vi "Vision Processing.vi"(4 "error in (no error)":errorcluster, 7 "Image Size":T1=enum."320x240") -> ()   [LabVIEW 2016]
doc: "This VI runs in parallel to other tasks. It gets images from the camera, processes them for color or shape and uses commands or globals to affect the behavior of other subsystems."
uses:
  <vilib>/Rock Robotics/WPI/Camera/WPI_CameraImageSize.ctl
  <vilib>/Rock Robotics/WPI/Camera/WPI_CameraWhite Balance Values.ctl
  <vilib>/Rock Robotics/WPI/Camera/WPI_CameraExposure Values.ctl
  <vilib>/Rock Robotics/WPI/Camera/WPI_CameraFrameRate.ctl
  Framework/Robot Global Data.vi
  Drive/Implementation/Drive Published Globals.vi
  <vilib>/Rock Robotics/Network Tables/NT Read Numeric Array.vi
  <vilib>/Rock Robotics/Network Tables/NT Write Number.vi
  <vilib>/Rock Robotics/Network Tables/NT Write Numeric Array.vi
  <vilib>/vision/NI_Vision_Development_Module.lvlib
panel:
  in  "Brightness":i32=20
  in  "Score Cutoff %":dbl=70.0
  in  "Particle Count Limit":dbl=inf
  out "Qualified Particles":i32=2
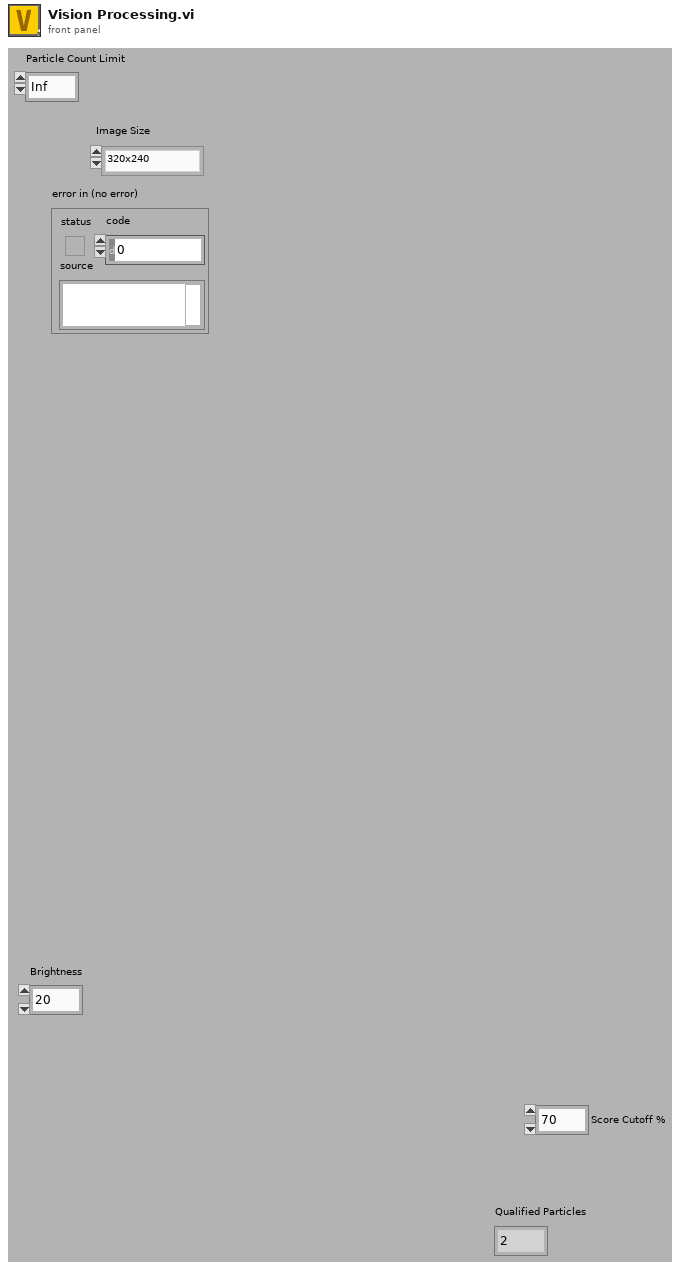
[diagram p1: front panel]
types:
  T1 = typedef "WPI_CameraImageSize.ctl" = enum16{"640x480", "320x240", "160x120", "Custom"}
  T2 = typedef "Image Type" = u32
  T3 = typedef "WPI_CameraFrameRate.ctl" = u32
  T4 = typedef "WPI_CameraExposure Values.ctl" = enum16{"Auto", "Flicker-free 50 Hz", "Flicker-free 60 Hz", "Hold current", "Custom"}
  T5 = typedef "WPI_CameraWhite Balance Values.ctl" = enum16{"Auto", "Fixed indoor", "Fixed outdoor 1", "Fixed outdoor 2", "Fixed fluorescent 1", "Fixed fluorescent 2", "Hold current", "Custom"}
  T6 = typedef "WPI_CameraDevRef.ctl" = cluster{"Camera Address":string, "CameraStatus":errorcluster}
  T7 = typedef "IMAQ Image.ctl" = refnum<image>
  T8 = cluster{"Left":dbl, "Top":dbl, "Right":dbl, "Bottom":dbl}
  T9 = typedef "Particle Parameters" = i32
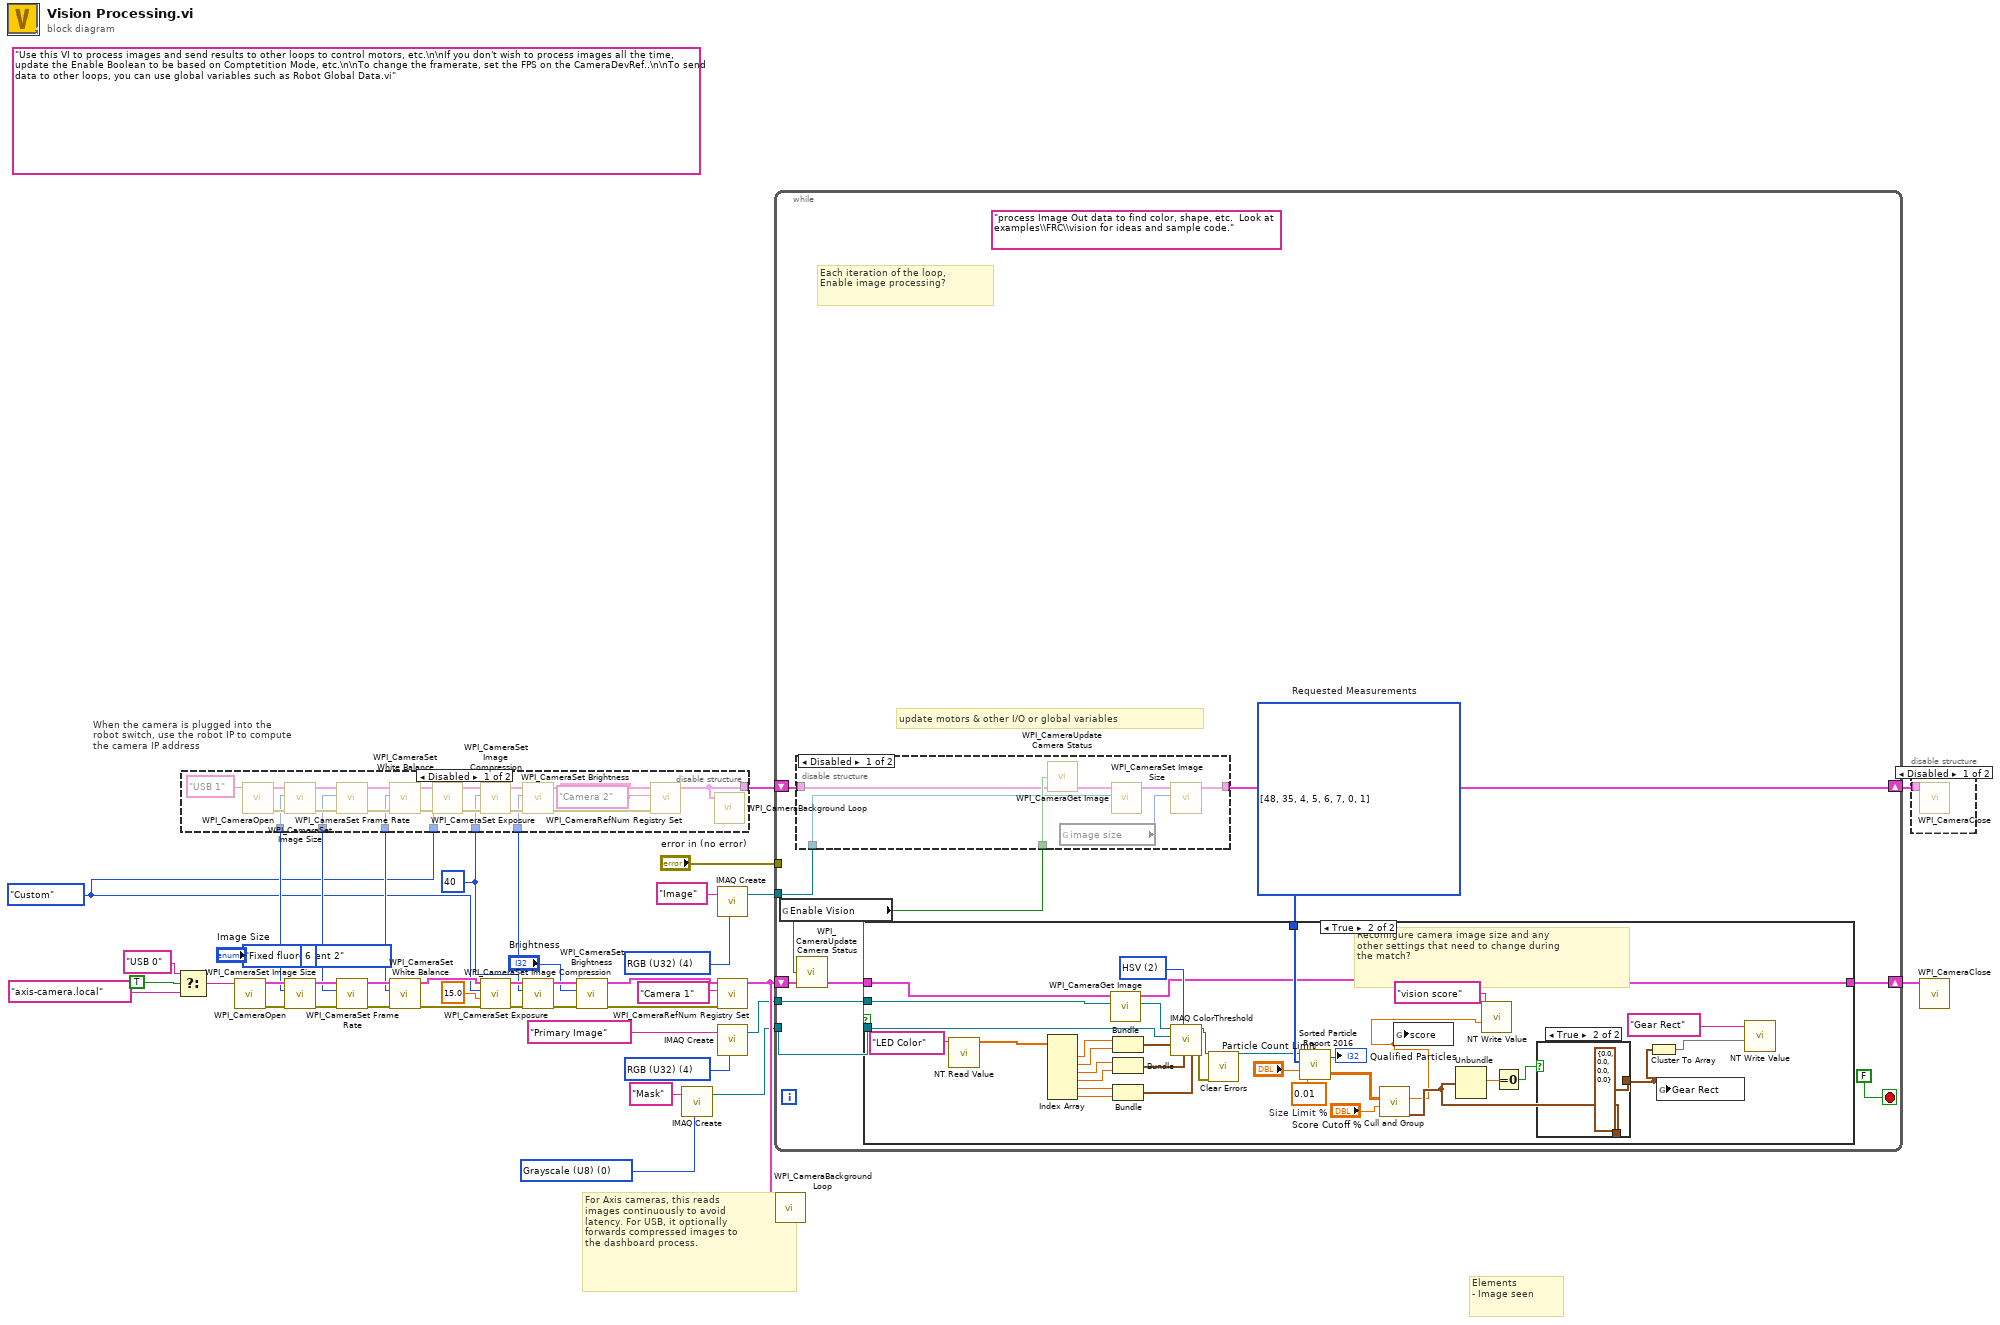
[diagram p0: block diagram]
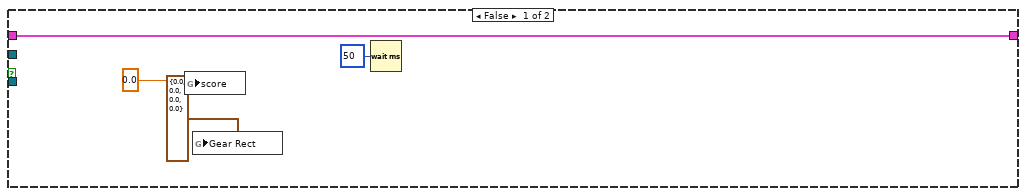
[diagram p4: hidden frame]
diagram:
  w3 = T2 0 items=["Grayscale (U8)", "Grayscale (I16)", "Grayscale (SGL)", "Complex (CSG)", "RGB (U32)", "HSL (U32)", "RGB (U64)", "Grayscale (U16)"] ("Image Type")
  w7 = T2 4 items=["Grayscale (U8)", "Grayscale (I16)", "Grayscale (SGL)", "Complex (CSG)", "RGB (U32)", "HSL (U32)", "RGB (U64)"] ("Image Type")
  w15 = T3 6 ("Frame Rate (fps)")
  w13 = WPI_CameraExposure_Values."Custom" ("Exposure")
  w14 = WPI_CameraWhite_Balance_Values."Fixed fluorescent 2" ("White Balance")
  w12 = 40 ("Compression")
  (unwired) "Use this VI to process images and send results to other loops to control motors, etc.\n\nIf you don't wish to process images all the time, update the Enable Boolean to be based on Comptetition Mode, etc.\n\nTo change the framerate, set the FPS on the CameraDevRef..\n\nTo send data to other loops, you can use global variables such as Robot Global Data.vi"
  w40 = T2 4 items=["Grayscale (U8)", "Grayscale (I16)", "Grayscale (SGL)", "Complex (CSG)", "RGB (U32)", "HSL (U32)", "RGB (U64)"] ("Image Type")
  # "Elements\n- Image seen"
  # "When the camera is plugged into the\nrobot switch, use the robot IP to compute\nthe camera IP address"
  # "For Axis cameras, this reads\nimages continuously to avoid\nlatency. For USB, it optionally\nforwards compressed images to\nthe dashboard process."
  n1 = Select(t="USB 0" ("format string"), s=TRUE ("dot notation? (F)"), f="axis-camera.local" ("format string")) -> (s? t:f=w18:string)
  n2 = disable-structure shown="Disabled" {
    disable-tunnel: "Image Size" -> [w48 _]
    disable-tunnel: w15 -> [w47 _]
    disable-tunnel: w14 -> [w46 _]
    disable-tunnel: w13 -> [w45 _]
    disable-tunnel: w12 -> [w44 _]
    disable-tunnel: "Brightness" -> [w43 _]
    disable-tunnel: [w41 _] -> w5
    frame Disabled {
      n3 = call <vilib>:"WPI_CameraOpen.vi"("Camera Address"="USB 1") -> ("error out"=w61:errorcluster, "CameraDevRef"=w62:T6)  [unwired: 2 in, 7 out]
      n4 = call <vilib>:"WPI_CameraSet Image Size.vi"("error in (no error)"=w61, "Image Size"=w48, "CameraDevRef"=w62) -> ("error out"=w54:errorcluster, "CameraDevRef Out"=w60:T6)  [unwired: 1 in, 6 out]
      n5 = call <vilib>:"WPI_CameraSet Frame Rate.vi"("error in (no error)"=w54, "Frame Rate (fps)"=w47, "CameraDevRef"=w60) -> ("error out"=w53:errorcluster, "CameraDevRef Out"=w59:T6)  [unwired: 7 out]
      n6 = call <vilib>:"WPI_CameraSet White Balance.vi"("error in (no error)"=w53, "White Balance"=w46, "CameraDevRef"=w59) -> ("error out"=w52:errorcluster, "CameraDevRef Out"=w58:T6)  [unwired: 1 in, 6 out]
      n7 = call <vilib>:"WPI_CameraSet Exposure.vi"("error in (no error)"=w52, "Exposure"=w45, "CameraDevRef"=w58) -> ("error out"=w51:errorcluster, "CameraDevRef Out"=w57:T6)  [unwired: 1 in, 6 out]
      n8 = call <vilib>:"WPI_CameraSet Image Compression.vi"("error in (no error)"=w51, "Compression"=w44, "CameraDevRef"=w57) -> ("error out"=w50:errorcluster, "CameraDevRef Out"=w56:T6)  [unwired: 7 out]
      n9 = call <vilib>:"WPI_CameraSet Brightness.vi"("error in (no error)"=w50, "Brightness"=w43, "CameraDevRef"=w56) -> ("error out"=w49:errorcluster, "CameraDevRef Out"=w55:T6)  [unwired: 7 out]
      n10 = call <vilib>:"WPI_CameraRefNum Registry Set.vi"("error in (no error)"=w49, "refnum name"="Camera 2", "CameraDevRef"=w55) -> ("CameraDevRef"=w41:T6)  [unwired: 1 in, 7 out]
      n11 = call <vilib>:"WPI_CameraBackground Loop.vi"("CameraDevRef"=w41) -> ()  [unwired: 11 in]
    }
    frame Enabled {
    }
  }
  n12 = call <vilib>:"WPI_CameraOpen.vi"("Camera Address"=w18) -> ("error out"=w31:errorcluster, "CameraDevRef"=w32:T6)  [unwired: 2 in, 7 out]
  n13 = call <vilib>:"WPI_CameraSet Image Size.vi"("error in (no error)"=w31, "Image Size"="Image Size", "CameraDevRef"=w32) -> ("error out"=w30:errorcluster, "CameraDevRef Out"=w33:T6)  [unwired: 1 in, 6 out]
  n14 = call <vilib>:"WPI_CameraSet Frame Rate.vi"("error in (no error)"=w30, "Frame Rate (fps)"=w15, "CameraDevRef"=w33) -> ("error out"=w29:errorcluster, "CameraDevRef Out"=w35:T6)  [unwired: 7 out]
  n15 = call <vilib>:"WPI_CameraSet White Balance.vi"("error in (no error)"=w29, "White Balance"=w14, "CameraDevRef"=w35) -> ("error out"=w28:errorcluster, "CameraDevRef Out"=w34:T6)  [unwired: 1 in, 6 out]
  n16 = call <vilib>:"WPI_CameraSet Exposure.vi"("error in (no error)"=w28, "Exposure (%)"=15.0, "Exposure"=w13, "CameraDevRef"=w34) -> ("error out"=w27:errorcluster, "CameraDevRef Out"=w37:T6)  [unwired: 6 out]
  n17 = call <vilib>:"WPI_CameraSet Image Compression.vi"("error in (no error)"=w27, "Compression"=w12, "CameraDevRef"=w37) -> ("error out"=w26:errorcluster, "CameraDevRef Out"=w36:T6)  [unwired: 7 out]
  n18 = call <vilib>:"WPI_CameraSet Brightness.vi"("error in (no error)"=w26, "Brightness"="Brightness", "CameraDevRef"=w36) -> ("error out"=w24:errorcluster, "CameraDevRef Out"=w25:T6)  [unwired: 7 out]
  n19 = call "IMAQ Create"("Image Name"="Mask", "Image Type"=w3) -> ("New Image"=w1:T7)  [unwired: 2 in, 2 out]
  n20 = call "IMAQ Create"("Image Name"="Image", "Image Type"=w7) -> ("New Image"=w6:T7)  [unwired: 2 in, 2 out]
  n21 = call <vilib>:"WPI_CameraRefNum Registry Set.vi"("error in (no error)"=w24, "refnum name"="Camera 1", "CameraDevRef"=w25) -> ("CameraDevRef"=w23:T6)  [unwired: 1 in, 7 out]
  n22 = call "IMAQ Create"("Image Name"="Primary Image", "Image Type"=w40) -> ("New Image"=w10:T7)  [unwired: 2 in, 2 out]
  n23 = while {
    shift-right: [w73] -> w22
    shift-left: w23 -> [w71]
    tunnel: w10 -> [w72]
    tunnel: "error in (no error)" -> [_]
    tunnel: w6 -> [w69]
    shift-right: [w68] -> w9
    shift-left: w5 -> [w67]
    tunnel: w1 -> [w66]
    stop <- FALSE stop-if-true
    w64 = T9[] [48, 35, 4, 5, 6, 7, 0, 1] items=["Center of Mass X", "Center of Mass Y", "First Pixel X", "First Pixel Y", "Bounding Rect Left", "Bounding Rect Top", "Bounding Rect Right", "Bounding Rect Bottom", "Max Feret Diameter Start X", "Max Feret Diameter Start Y", "Max Feret Diameter End X", "Max Feret Diameter End Y", "Max Horiz. Segment Length Left", "Max Horiz. Segment Length Right", "Max Horiz. Segment Length Row", "-", "Bounding Rect Width", "Bounding Rect Height", "Bounding Rect Diagonal", "Perimeter", "Convex Hull Perimeter", "Holes' Perimeter", "Max Feret Diameter", "Equivalent Ellipse Major Axis", "Equivalent Ellipse Minor Axis", "Equivalent Ellipse Minor Axis (Feret)", "Equivalent Rect Long Side", "Equivalent Rect Short Side", "Equivalent Rect Diagonal", "Equivalent Rect Short Side (Feret)", "Average Horiz. Segment Length", "Average Vert. Segment Length", "Hydraulic Radius", "Waddel Disk Diameter", "-", "Area", "Holes' Area", "Particle & Holes' Area", "Convex Hull Area", "Image Area", "-", "Number of Holes", "Number of Horiz. Segments", "Number of Vert. Segments", "-", "Orientation", "Max Feret Diameter Orientation", "-", "% Area/Image Area", "% Area/(Particle & Holes' Area)", "Ratio of Equivalent Ellipse Axes", "Ratio of Equivalent Rect Sides", "-", "Elongation Factor", "Compactness Factor", "Heywood Circularity Factor", "Type Factor", "-", "Sum X", "Sum Y", "Sum XX", "Sum XY", "Sum YY", "Sum XXX", "Sum XXY", "Sum XYY", "Sum YYY", "-", "Moment of Inertia XX", "Moment of Inertia XY", "Moment of Inertia YY", "Moment of Inertia XXX", "Moment of Inertia XXY", "Moment of Inertia XYY", "Moment of Inertia YYY", "Norm. Moment of Inertia XX", "Norm. Moment of Inertia XY", "Norm. Moment of Inertia YY", "Norm. Moment of Inertia XXX", "Norm. Moment of Inertia XXY", "Norm. Moment of Inertia XYY", "Norm. Moment of Inertia YYY", "Hu Moment 1", "Hu Moment 2", "Hu Moment 3", "Hu Moment 4", "Hu Moment 5", "Hu Moment 6", "Hu Moment 7"]  # Requested Measurements
    (unwired) "process Image Out data to find color, shape, etc.  Look at examples\\FRC\\vision for ideas and sample code."
    # "update motors & other I/O or global variables"
    # "Each iteration of the loop,\nEnable image processing?"
    n24 = global read "Robot Global Data.vi" "Enable Vision"() -> (w65:bool)
    n25 = disable-structure shown="Disabled" {
      disable-tunnel: w65 -> [w120 _]
      disable-tunnel: w69 -> [w118 _]
      disable-tunnel: [w117 _] -> w68
      disable-tunnel: w67 -> [w116 _]
      frame Disabled {
        n26 = call <vilib>:"WPI_CameraUpdate Camera Status.vi"("CameraDevRef In"=w116, "Enable Vision"=w120) -> ("CameraDevRef Out"=w119:T6)  [unwired: 3 in]
        n27 = global read "Robot Global Data.vi" "image size"() -> (w115:T1)
        n28 = call <vilib>:"WPI_CameraGet Image.vi"("Image"=w118, "CameraDevRef"=w119) -> ("CameraDevRef Out"=w114:T6)  [unwired: 1 in, 8 out]
        n29 = call <vilib>:"WPI_CameraSet Image Size.vi"("Image Size"=w115, "CameraDevRef"=w114) -> ("CameraDevRef Out"=w117:T6)  [unwired: 2 in, 7 out]
      }
      frame Enabled {
      }
    }
    n30 = call <vilib>:"WPI_CameraUpdate Camera Status.vi"("CameraDevRef In"=w71, "Enable Vision"=w65) -> ("CameraDevRef Out"=w70:T6)  [unwired: 3 in]
    n31 = case shown="True" w65 {
      tunnel: [w78 w83] -> w73
      tunnel: w72 -> [_ w111]
      tunnel: w70 -> [w78 w110]
      tunnel: w66 -> [_ w108]
      tunnel: w64 -> [_ w91]
      frame False {
        n32 = global write "Drive Published Globals.vi" "score"(0.0) -> ()
        n33 = global write "Drive Published Globals.vi" "Gear Rect"(T8 {"Left"=0.0, "Top"=0.0, "Right"=0.0, "Bottom"=0.0} ("Gear Rect")) -> ()
        n34 = Wait (ms)(milliseconds to wait=u32 50) -> ()  [unwired: 1 out]
      }
      frame True {
        w92 = u16 2 items=["RGB", "HSL", "HSV", "HSI"] ("Color Mode")
        w95 = 0.01  # Size Limit %
        # "Reconfigure camera image size and any\nother settings that need to change during\nthe match?"
        n35 = call-poly <vilib>:"NT Read Value.vi"("Name"="LED Color") -> ("Numeric Array"=w106:dbl[])  [unwired: 9 in, 1 out]
        n36 = Index Array(array=w106) -> (element #1=w104:dbl, element #2=w105:dbl, element #3=w103:dbl, element #4=w102:dbl, element #5=w101:dbl, element #6=w100:dbl)  [unwired: 6 in]
        n37 = call <vilib>:"WPI_CameraGet Image.vi"("Image"=w111, "CameraDevRef"=w110) -> ("Image Out"=w109:T7, "CameraDevRef Out"=w83:T6)  [unwired: 1 in, 7 out]
        n38 = Bundle("Numeric"=w104, "Numeric"=w105) -> (w99:cluster{"Numeric":dbl, "Numeric":dbl})  [unwired: 1 in]
        n39 = Bundle("Numeric"=w103, "Numeric"=w102) -> (w98:cluster{"Numeric":dbl, "Numeric":dbl})  [unwired: 1 in]
        n40 = Bundle("Numeric"=w101, "Numeric"=w100) -> (w97:cluster{"Numeric":dbl, "Numeric":dbl})  [unwired: 1 in]
        n41 = call "IMAQ ColorThreshold"("Blue or Luma or Val or Inten Range"=w97, "Green or Sat Range"=w98, "Color Mode"=w92, "Red or Hue Range"=w99, "Image Dst"=w108, "Image Src"=w109) -> ("error out"=w96:errorcluster, "Image Dst Out"=w87:T7)  [unwired: 4 in]
        n42 = call <vilib>:"Clear Errors.vi"("error in (no error)"=w96) -> ()  [unwired: 5 in, 2 out]
        n43 = call "Sorted Particle Report 2016.vi"("Min Area Size %"=w95, "Particle Count Limit"="Particle Count Limit", "Pixel Measurements"=w91, "Image in"=w87) -> ("Sorted Data"=w81:dbl[][], "Particles"=→"Qualified Particles":i32)
        n44 = call "Cull and Group.vi"("Score Cutoff"="Score Cutoff %", "Sorted Data"=w81) -> ("Rect"=w80:T8, "Score"=w79:dbl)  [unwired: 6 in, 2 out]
        n45 = global write "Drive Published Globals.vi" "score"(w79) -> ()
        n46 = Unbundle(w80) -> ("Top"=w89:dbl)  [unwired: 3 out]
        n47 = call-poly <vilib>:"NT Write Value.vi"("Numeric"=w79, "Name"="vision score") -> ()  [unwired: 9 in, 1 out]
        n48 = Equal To 0?(x=w89) -> (x = 0?=w88:bool)
        n49 = case shown="True" w88 {
          tunnel: [w112 T8 {"Left"=0.0, "Top"=0.0, "Right"=0.0, "Bottom"=0.0} ("Rect")] -> w86
          tunnel: w80 -> [w112 _]
          frame False {
          }
          frame True {
          }
        }
        n50 = Cluster To Array(cluster=w86) -> (array=w84:dbl[])
        n51 = global write "Drive Published Globals.vi" "Gear Rect"(w86) -> ()
        n52 = call-poly <vilib>:"NT Write Value.vi"("Numeric Array"=w84, "Name"="Gear Rect") -> ()  [unwired: 9 in, 1 out]
      }
    }
  }
  n53 = call <vilib>:"WPI_CameraBackground Loop.vi"("CameraDevRef"=w23) -> ()  [unwired: 11 in]
  n54 = disable-structure shown="Disabled" {
    disable-tunnel: w9 -> [w121 _]
    frame Disabled {
      n55 = call <vilib>:"WPI_CameraClose.vi"("CameraDevRef"=w121) -> ()  [unwired: 1 in, 10 out]
    }
    frame Enabled {
    }
  }
  n56 = call <vilib>:"WPI_CameraClose.vi"("CameraDevRef"=w22) -> ()  [unwired: 1 in, 10 out]
